vi "pc_write_cond.vi"(0 "X":dbl[](array[numeric]), 1 "Y":dbl[](array[numeric]), 2 "Auto Dispense Flag":bool[](array[boolean]), 3 "Touch 1":bool[](array[boolean]), 4 "Touch 2":bool[](array[boolean]), 5 "Nose Poke":bool[](array[boolean]), 6 "Acquire On":bool, 7 "Dispense":bool[](array[boolean]), 9 "Trial Live":bool[](array[boolean]), 10 "Count In":i32, 11 "Opto On":bool[](array[boolean]), 12 "Max Count":i32=2, 13 "Lick":bool[](array[boolean])) -> (14 "Write Current":bool, 15 "Write Previous":bool, 17 "Current Data":string, 18 "Previous Data":string, 19 "Count Out":i32)   [LabVIEW 2013]
doc: "Convert individual time series arrays of sensor readings into a strings. Each line in the output string represents all the sensor readings for one time step.\n\nAlso, decide whether to write previous data, write current data, and what value to give Count Out"
panel:
  out "size(s)":i32
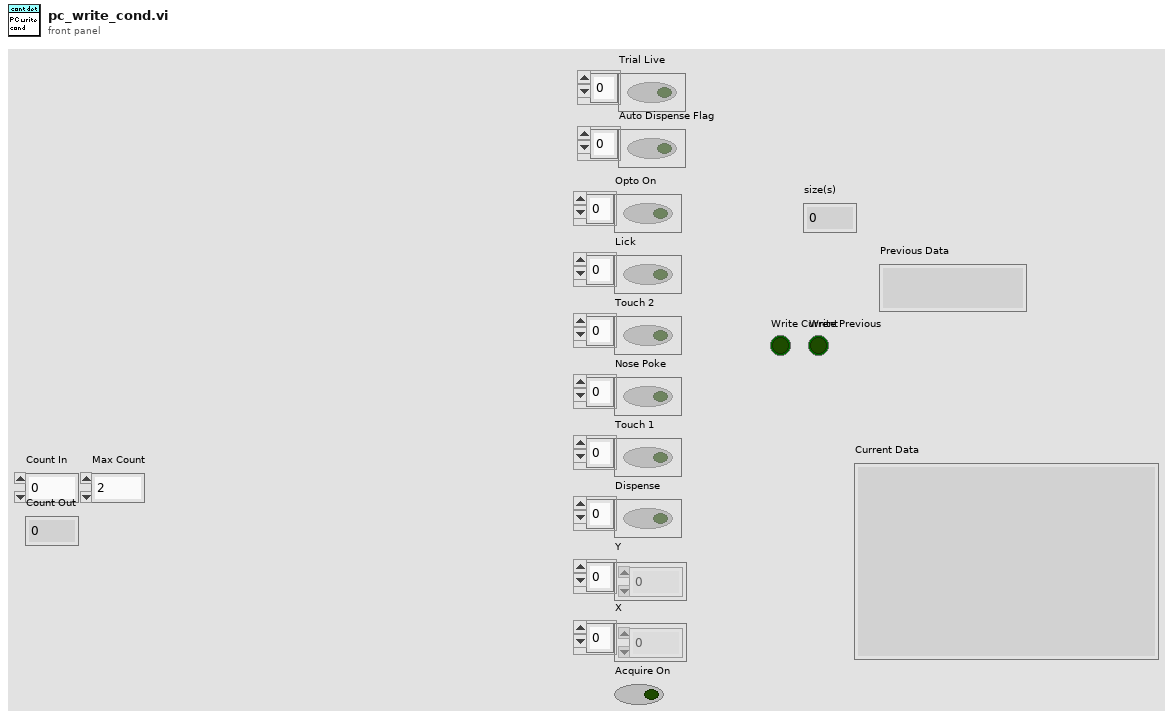
[diagram p1: front panel]
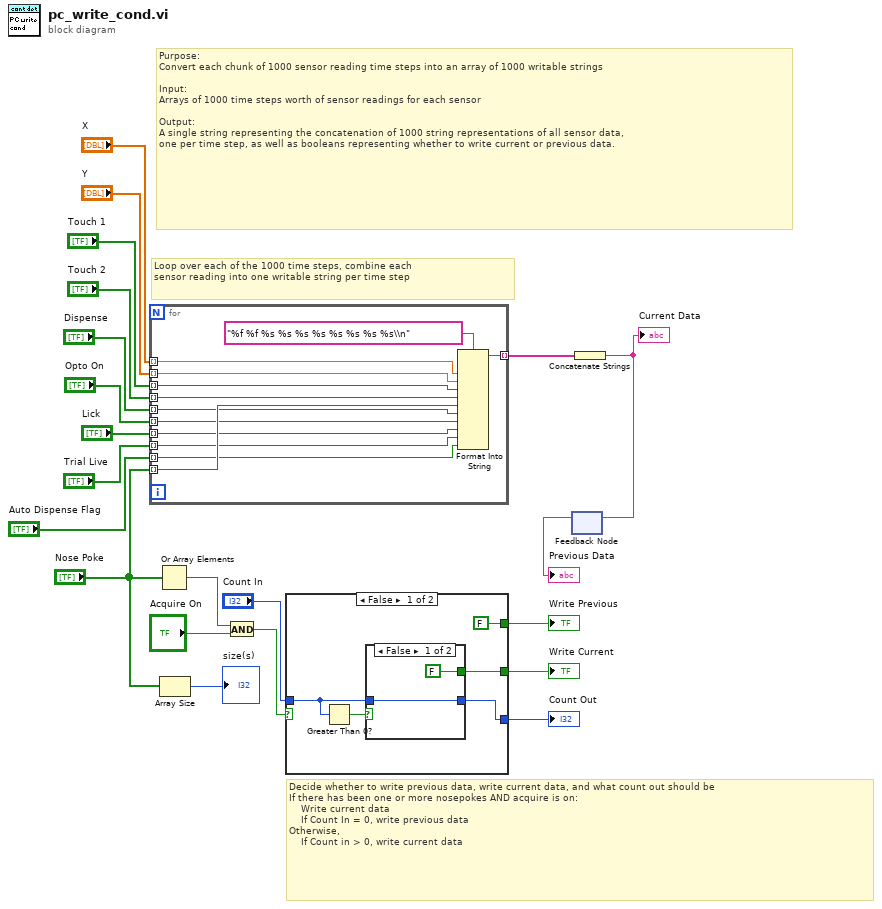
[diagram p0: block diagram]
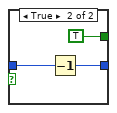
[diagram p2: hidden frame]
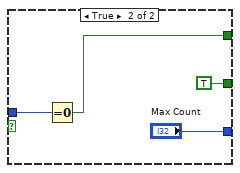
[diagram p3: hidden frame]
diagram:
  # "Purpose:\nConvert each chunk of 1000 sensor reading time steps into an array of 1000 writable strings\n\nInput:\nArrays of 1000 time steps worth of sensor readings for each sensor\n\nOutput:\nA single string representing the concatenation of 1000 string representations of all sensor data, \none per time step, as well as booleans representing whether to write current or previous data."
  # "Loop over each of the 1000 time steps, combine each \nsensor reading into one writable string per time step"
  # "Decide whether to write previous data, write current data, and what count out should be\nIf there has been one or more nosepokes AND acquire is on:\n    Write current data\n    If Count In = 0, write previous data\nOtherwise,\n    If Count in > 0, write current data"
  n1 = for {
    tunnel: "X" -> [w33] mode=indexing
    tunnel: "Y" -> [w32] mode=indexing
    tunnel: "Touch 1" -> [w31] mode=indexing
    tunnel: "Touch 2" -> [w30] mode=indexing
    tunnel: "Nose Poke" -> [w29] mode=indexing
    tunnel: "Dispense" -> [w28] mode=indexing
    tunnel: [w26] -> w15 mode=indexing
    tunnel: "Opto On" -> [w25] mode=indexing
    tunnel: "Lick" -> [w24] mode=indexing
    tunnel: "Trial Live" -> [w23] mode=indexing
    tunnel: "Auto Dispense Flag" -> [w22] mode=indexing
    n2 = Format Into String(format string="%f %f %s %s %s %s %s %s %s %s\\n", w33, w32, w31, w30, w29, w28, w25, w24, w23, w22) -> (resulting string=w26:string)  [unwired: 2 in, 1 out]
  }
  n3 = Or Array Elements(Boolean array="Nose Poke") -> (logical OR=w4:bool)
  n4 = Array Size(array="Nose Poke") -> (size(s)=→"size(s)":i32)
  n5 = And(x=w4, y="Acquire On") -> (x .and. y?=w5:bool)
  n6 = case shown="False" w5 {
    tunnel: "Count In" -> [w37 w47]
    tunnel: [w36 "Max Count"] -> w12
    tunnel: [FALSE w45] -> w11
    tunnel: [w35 TRUE] -> w10
    frame False {
      n7 = Greater Than 0?(x=w37) -> (x > 0?=w38:bool)
      n8 = case shown="False" w38 {
        tunnel: w37 -> [w40 w43]
        tunnel: [w40 w42] -> w36
        tunnel: [FALSE TRUE] -> w35
        frame False {
        }
        frame True {
          n9 = Decrement(x=w43) -> (x-1=w42:i32)
        }
      }
    }
    frame True {
      n10 = Equal To 0?(x=w47) -> (x = 0?=w45:bool)
    }
  }
  "Write Current" <- w10
  "Count Out" <- w12
  "Write Previous" <- w11
  n11 = feedback #1() -> (→"Previous Data":string)  [unwired: 1 in]
  n12 = Concatenate Strings(w15) -> (w14:string)
  "Current Data" <- w14
  n13 = feedback-in #1(w14) -> ()
